vi "Is Over-Range.vi"(8 "error in (no error)":errorcluster, 10 "measurement value":dbl format="%^.2e", 11 "IVI_DMM in":refnum<class "IVI_DMM.lvclass">) -> (0 "error out":errorcluster, 2 "is over-range":bool, 3 "IVI_DMM out":refnum<class "IVI_DMM.lvclass">)   [LabVIEW 2013, in "IVI_DMM.lvlib" / "IVI_DMM.lvclass"]
doc: "This VI takes a measurement value that you obtain from either the Read or Fetch VIs and determines if the value is a valid measurement value or a value indicating that an over-range condition occurred. \n\nNotes:\n\n(1) If an over-range condition occurs, the measurement value contains an IEEE defined NaN (Not a Number) value indicating that an over-range condition occurred.\n\n(2) This VI does not check the instrument status."
uses:
  IVI_DMM.lvclass
  IVI_DMM.lvclass/IVI_DMM.ctl
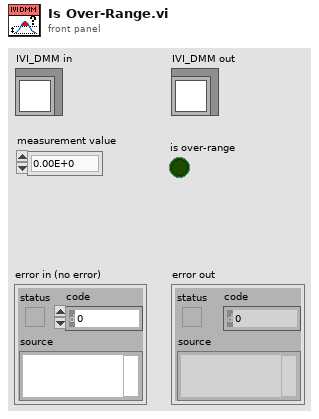
[diagram p1: front panel]
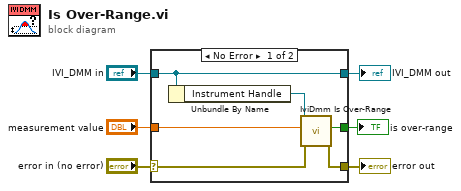
[diagram p0: block diagram]
diagram:
  n1 = case shown="No Error" "error in (no error)" {
    selector: "error in (no error)" -> [w10 w14]
    tunnel: [w9 w14] -> w5
    tunnel: [w12 w13] -> w3
    tunnel: "IVI_DMM in" -> [w12 w13]
    tunnel: [w8 _] -> w2
    tunnel: "measurement value" -> [w7 _]
    frame No Error {
      n2 = Unbundle By Name(w12) -> ("Instrument Handle"=w11:refnum<k15>)
      n3 = call <vilib>:"IviDmm Is Over-Range.vi"("error in (no error)"=w10, "measurement value"=w7, "instrument handle"=w11) -> ("error out"=w9:errorcluster, "is over-range"=w8:bool)  [unwired: 6 in, 1 out]
    }
    frame Error {
    }
  }
  "error out" <- w5
  "IVI_DMM out" <- w3
  "is over-range" <- w2
